vi "adsorption_rig_main.vi"() -> ()   [LabVIEW 2020]
uses:
  adam5000_LLB/controls/adam-5000-serial-settings.ctl
  adam5000_LLB/controls/adam-5000-cmd-response.ctl
  adam5000_LLB/controls/state-enum.ctl
  adam5000_LLB/sub-vi/csv-file-logging/filepath-selection.ctl
  adam5000_LLB/controls/adam-5000-all-chassis-data.ctl
  adam5000_LLB/controls/adam-5000-all-module-datas.ctl
  adam5000_LLB/controls/digital-output-cluster.ctl
  adam5000_LLB/controls/digitial-input-cluster.ctl
  adam5000_LLB/controls/analog-output-cluster.ctl
  adam5000_LLB/controls/analog-input-cluster.ctl
  adam5000_LLB/controls/thermocouple-input-cluster.ctl
  adam5000_LLB/controls/adam-5000-chassis-cmd-ack.ctl
  adam5000_LLB/controls/adam-5000-chassis-module-types.ctl
  adam5000_LLB/controls/adam-5000-DO-user-input.ctl
  adam5000_LLB/controls/adam-5000-status-indicator-references.ctl
panel:
  in  "Reset LD":bool
  out "longest delay":u32
  out "Next Log Event mS":u32
  in  "Tab Control":enum32{"System", "Settings"}(tab)
  in  "Flow 4":dbl
  in  "Flow 3":dbl
  in  "Flow 2":dbl
  in  "Flow 1":dbl
  in  "V9: EP1":bool
  in  "V12: EP4":bool
  in  "V10: EP2":bool
  in  "V11: EP3":bool
  in  "V15: \nRecirculation":bool
  in  "V14: HR2":bool
  out "TC9":dbl
  in  "V13: HR1":bool
  out "TC8":dbl
  in  "V8: In4":bool
  out "TC1":dbl
  out "TC2":dbl
  out "TC3":dbl
  out "TC4":dbl
  out "TC5":dbl
  out "TC6":dbl
  out "TC7":dbl
  out "TC10":dbl
  out "TC11":dbl
  out "TC12":dbl
  in  "V1: Ex1":bool
  in  "V2: Ex2":bool
  in  "V4: Ex4":bool
  in  "V5: In1":bool
  in  "V6: In2":bool
  in  "V7: In3":bool
  out "P1: Condenser":dbl
  out "P2: Adsorber 2":dbl
  out "P3: Adsorber 1":dbl
  out "P4: Evaporator":dbl
  in  "V3: Ex3":bool
  in  "Additional CSV Data Heading":string="Flow1,Flow2,Flow3,Flow4"
  in  "Chassis Settings":T1={"VISA resource name"="COM4", "baud rate (19200)"=19200, "Chassis ID"=1}
  in  "Log Filepath Selection":T2={"Log Filepath Source"=enum."Application Relative (Auto)", "Log File Path (Manual)"=path "C:/Users/iwheard/Documents/0000-labview/adam5000-generic-controller/data", "Log File Folder Name"="data", "log file name"="log", "Include Date in Filename"=TRUE, "Include Time in Filename"=TRUE}
  out "Log Filepath":path
  out "log start time":u32
  out "log-elapsed time":dbl format="%.2f"
  in  "CSV Data Headings":string="time (s),T1,T2,T3,T4,T5,T6,T7,T8,T9,T10,T11,T12,P1,P2,P3,P4"
  out "Logged Data String":string
  out "error":errorcluster
  out "Hz":dbl format="%_3g"
  in  "Sample Rate (Hz)":dbl=1.0 min=0.0001 max=4.0 format="%#_4g"
  out "File Open":bool
  out "Logging Active":bool
  out "Error Detected":bool
  in  "Reset":bool
  out "ADAM Connected":bool
  in  "Stop ADAM":bool
  in  "Start Logging":bool
  out "Program State":T3
  in  "Start ADAM":bool
  out "cmd-response":T5
  out "Status Indicators":T6
  in  "Debug Mode":bool
  out "Loop Time (mS)":u32
  out "Loop Counter":i32
  in  "exit":bool
  # "Adsorption Rig 2025"
  # "Built By: \nImogen Heard"
  # "Cold"
  # "Ambient"
  # "Hot"
  # "NV-002"
  # "NV-001"
  # "NV-004"
  # "Flow 4"
  # "Flow 1"
  # "Flow 2"
  # "NV-003"
  # "Flow 3"
  # "Condenser"
  # "Adsorber 1"
  # "Adsorber 2"
  # "Evaporator"
  # "Flow Meter Inputs"
  # "Pressure Sensors"
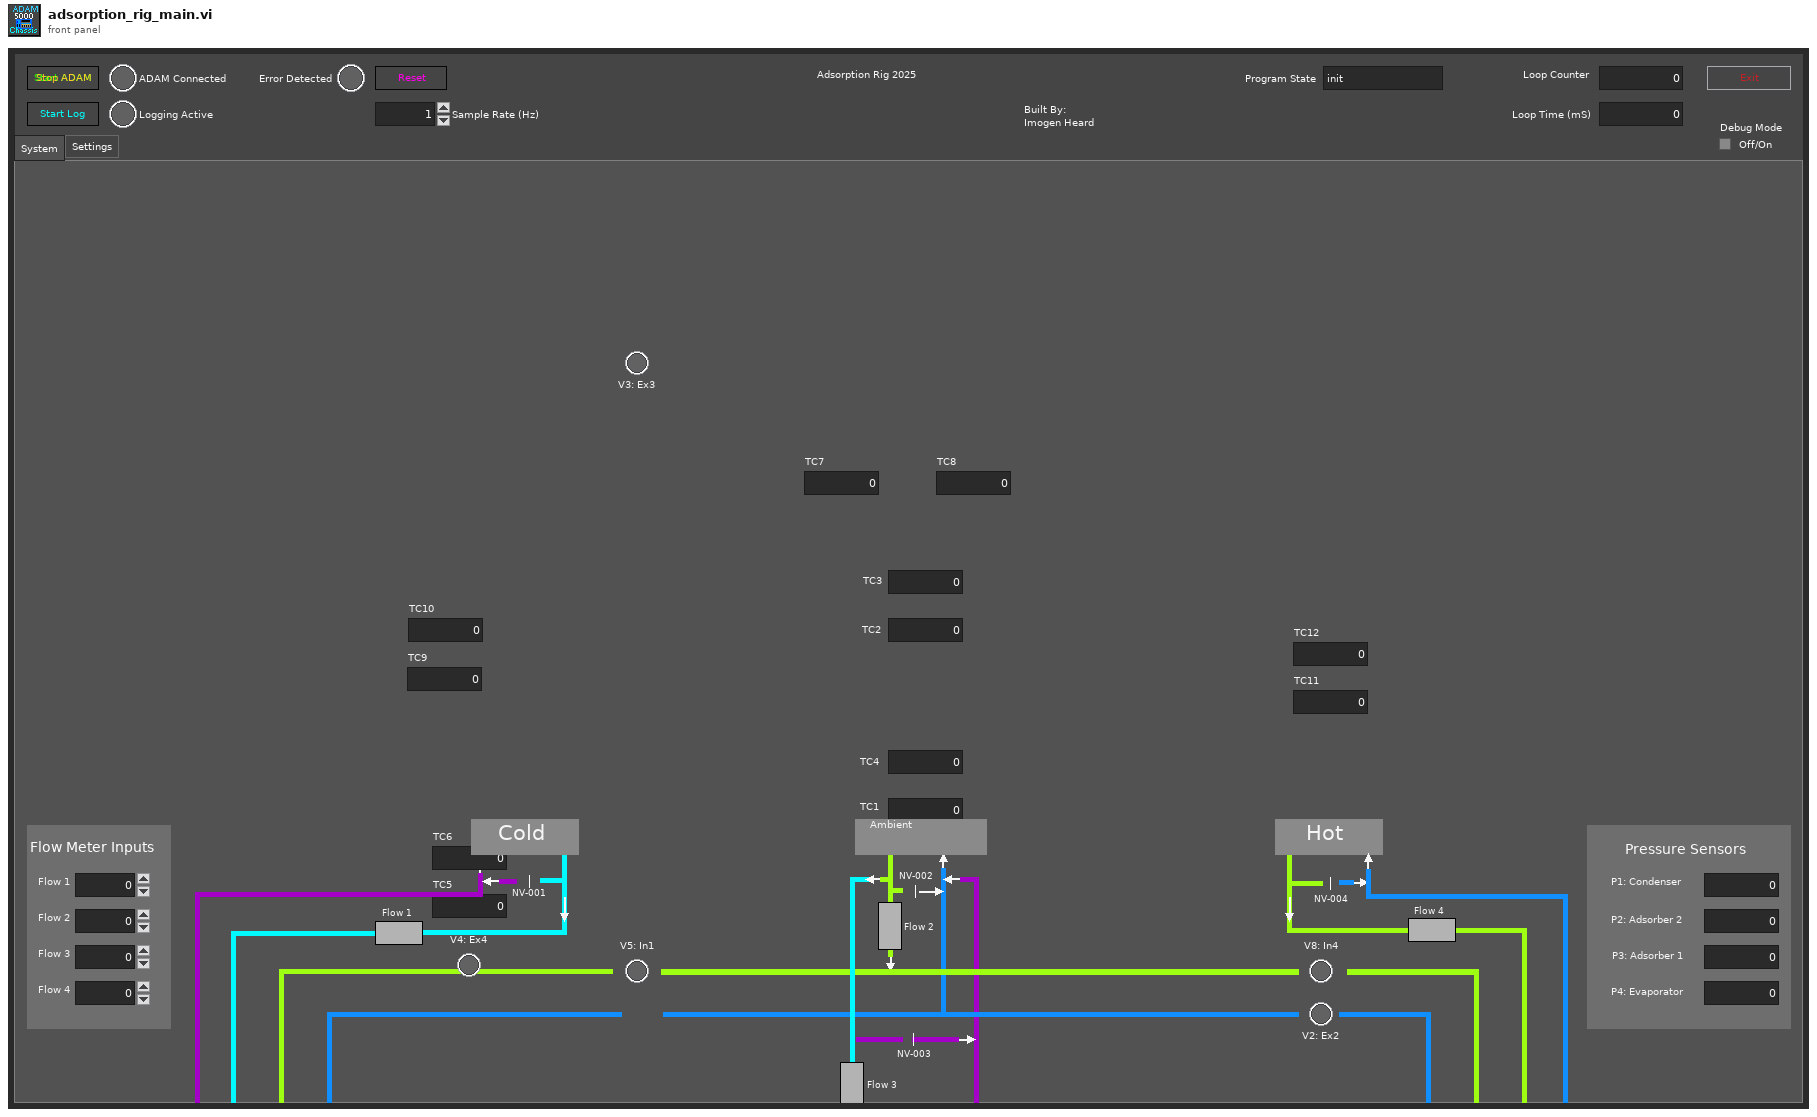
[diagram p1: front panel]
types:
  T1 = typedef "adam-5000-serial-settings.ctl" = cluster{"VISA resource name":refnum<visa-resource-name>, "baud rate (19200)":u32, "Chassis ID":u8}
  T2 = typedef "filepath-selection.ctl" = cluster{"Log Filepath Source":enum16{"Application Relative (Auto)", "VI Relative (Auto)", "Complete Path (Manual)"}, "Log File Path (Manual)":path, "Log File Folder Name":string, "log file name":string, "Include Date in Filename":bool, "Include Time in Filename":bool}
  T3 = typedef "state-enum.ctl" = enum16{"init", "wait", "manual", "start", "run", "reset", "stop", "exit"}
  T4 = typedef "adam-5000-cmd-response.ctl" = cluster{"cmd string":string, "response":string}
  T5 = cluster{"cmd-response:0":T4, "cmd-response:1":T4, "cmd-response:2":T4, "cmd-response:3":T4, "cmd-response:4":T4, "cmd-response:5":T4, "cmd-response:6":T4, "cmd-response:7":T4}
  T6 = cluster{"status-indicator:0":cluster{"Sampling":bool, "Ack":bool}, "status-indicator:1":cluster{"Sampling":bool, "Ack":bool}, "status-indicator:2":cluster{"Sampling":bool, "Ack":bool}, "status-indicator:3":cluster{"Sampling":bool, "Ack":bool}, "status-indicator:4":cluster{"Sampling":bool, "Ack":bool}, "status-indicator:5":cluster{"Sampling":bool, "Ack":bool}, "status-indicator:6":cluster{"Sampling":bool, "Ack":bool}, "status-indicator:7":cluster{"Sampling":bool, "Ack":bool}}
  T7 = enum16{"Digital Output", "Digital Input", "Analog Output", "Analog Input", "Thermocouple", "Power Relay", "empty"}
  T8 = typedef "adam-5000-chassis-module-types.ctl" = cluster{"Slot 0: Module Type":enum16{"Digital Output", "Digital Input", "Analog Output", "Analog Input", "Thermocouple", "Power Relay", "empty"}, "Slot 1: Module Type":enum16{"Digital Output", "Digital Input", "Analog Output", "Analog Input", "Thermocouple", "Power Relay", "empty"}, "Slot 2: Module Type":enum16{"Digital Output", "Digital Input", "Analog Output", "Analog Input", "Thermocouple", "Power Relay", "empty"}, "Slot 3: Module Type":enum16{"Digital Output", "Digital Input", "Analog Output", "Analog Input", "Thermocouple", "Power Relay", "empty"}, "Slot 4: Module Type":enum16{"Digital Output", "Digital Input", "Analog Output", "Analog Input", "Thermocouple", "Power Relay", "empty"}, "Slot 5: Module Type":enum16{"Digital Output", "Digital Input", "Analog Output", "Analog Input", "Thermocouple", "Power Relay", "empty"}, "Slot 6: Module Type":enum16{"Digital Output", "Digital Input", "Analog Output", "Analog Input", "Thermocouple", "Power Relay", "empty"}, "Slot 7: Module Type":enum16{"Digital Output", "Digital Input", "Analog Output", "Analog Input", "Thermocouple", "Power Relay", "empty"}}
  T9 = typedef "adam-5000-chassis-cmd-ack.ctl" = cluster{"cmd-response:0":T4, "cmd-response:1":T4, "cmd-response:2":T4, "cmd-response:3":T4, "cmd-response:4":T4, "cmd-response:5":T4, "cmd-response:6":T4, "cmd-response:7":T4}
  T10 = typedef "adam-5000-all-chassis-data.ctl" = cluster{"slot:0":T11, "slot:1":T11, "slot:2":T11, "slot:3":T11, "slot:4":T11, "slot:5":T11, "slot:6":T11, "slot:7":T11}
  T11 = typedef "adam-5000-all-module-datas.ctl" = cluster{"Digital Outputs":T12, "Digital Inputs":T13, "Analog Outputs":T14, "Analog Inputs":T15, "Thermocouple Inputs (degC)":T16}
  T12 = typedef "digital-output-cluster.ctl" = cluster{"DO0":bool, "DO1":bool, "DO2":bool, "DO3":bool, "DO4":bool, "DO5":bool, "DO6":bool, "DO7":bool}
  T13 = typedef "digitial-input-cluster.ctl" = cluster{"DI0":bool, "DI1":bool, "DI2":bool, "DI3":bool, "DI4":bool, "DI5":bool, "DI6":bool, "DI7":bool}
  T14 = typedef "analog-output-cluster.ctl" = cluster{"AO0":dbl, "AO1":dbl, "AO2":dbl, "AO3":dbl}
  T15 = typedef "analog-input-cluster.ctl" = cluster{"AI0":dbl, "AI1":dbl, "AI2":dbl, "AI3":dbl, "AI4":dbl, "AI5":dbl, "AI6":dbl, "AI7":dbl}
  T16 = typedef "thermocouple-input-cluster.ctl" = cluster{"TC0":dbl, "TC1":dbl, "TC2":dbl, "TC3":dbl, "TC4":dbl, "TC5":dbl, "TC6":dbl}
  T17 = enum8{"Enabled", "Disabled", "Disabled and Grayed Out"}
  T18 = typedef "adam-5000-status-indicator-references.ctl" = cluster{"status-indicator:0":refnum<vi>, "status-indicator:1":refnum<vi>, "status-indicator:2":refnum<vi>, "status-indicator:3":refnum<vi>, "status-indicator:4":refnum<vi>, "status-indicator:5":refnum<vi>, "status-indicator:6":refnum<vi>, "status-indicator:7":refnum<vi>}
  T19 = typedef "adam-5000-DO-user-input.ctl" = cluster{"0:Digital Outputs":T12, "1:Digital Outputs":T12, "2:Digital Outputs":T12, "3:Digital Outputs":T12, "4:Digital Outputs":T12, "5:Digital Outputs":T12, "6:Digital Outputs":T12, "7:Digital Outputs":T12}
  T20 = cluster{"V1: Ex1":bool, "V2: Ex2":bool, "V3: Ex3":bool, "V4: Ex4":bool, "V5: In1":bool, "V6: In2":bool, "V7: In3":bool, "V8: In4":bool}
  T21 = cluster{"V9: EP1":bool, "V10: EP2":bool, "V11: EP3":bool, "V12: EP4":bool, "V13: HR1":bool, "V14: HR2":bool, "V15: \nRecirculation":bool, "V9: EP1":bool}
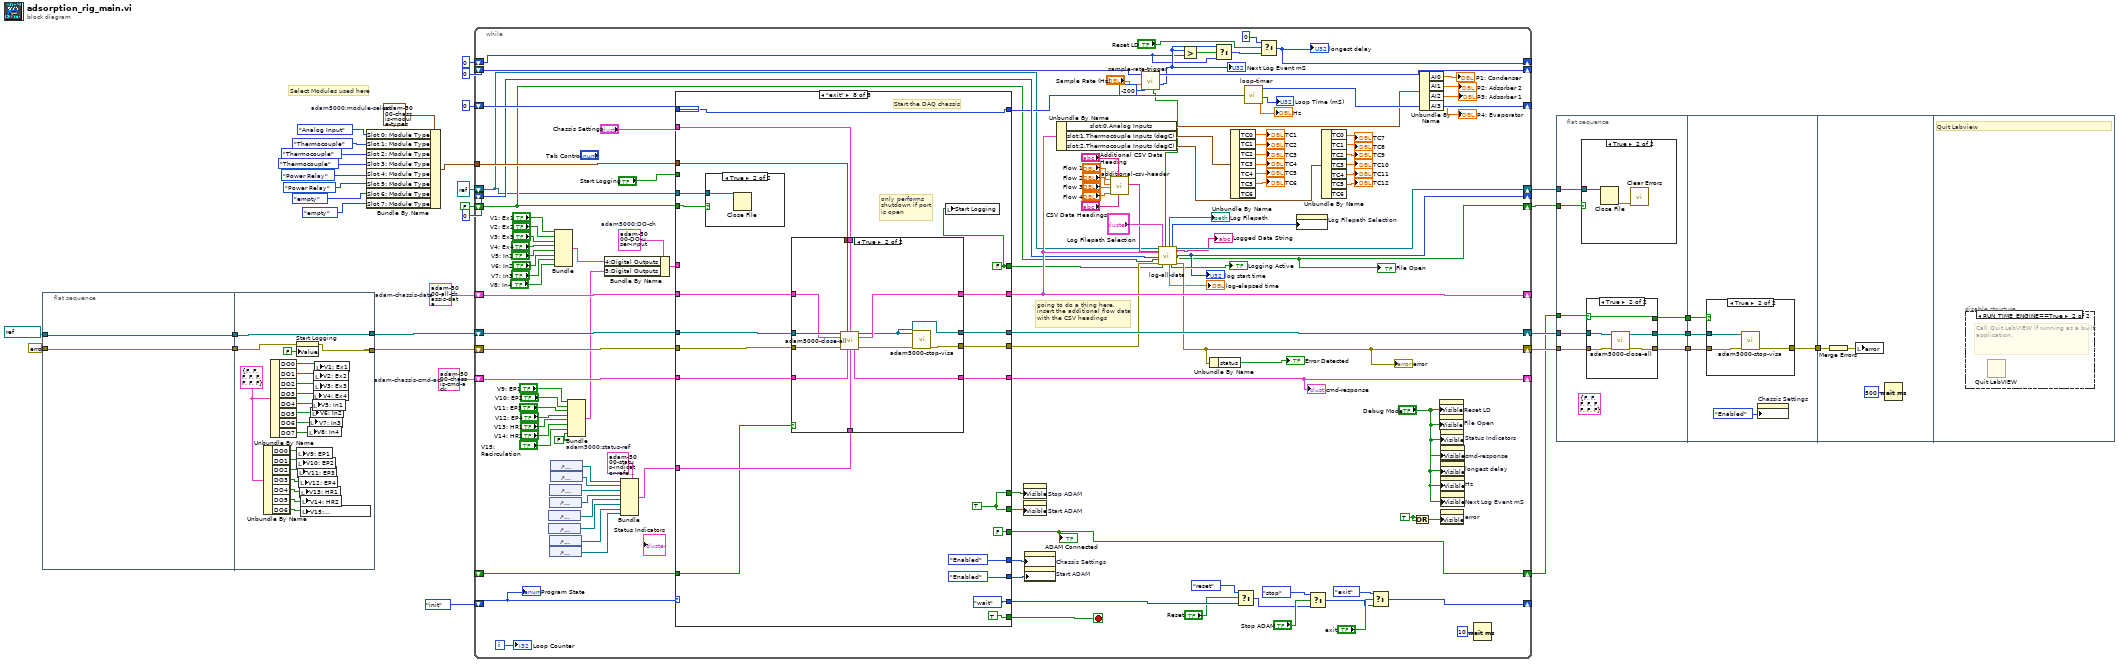
[diagram p0: block diagram]
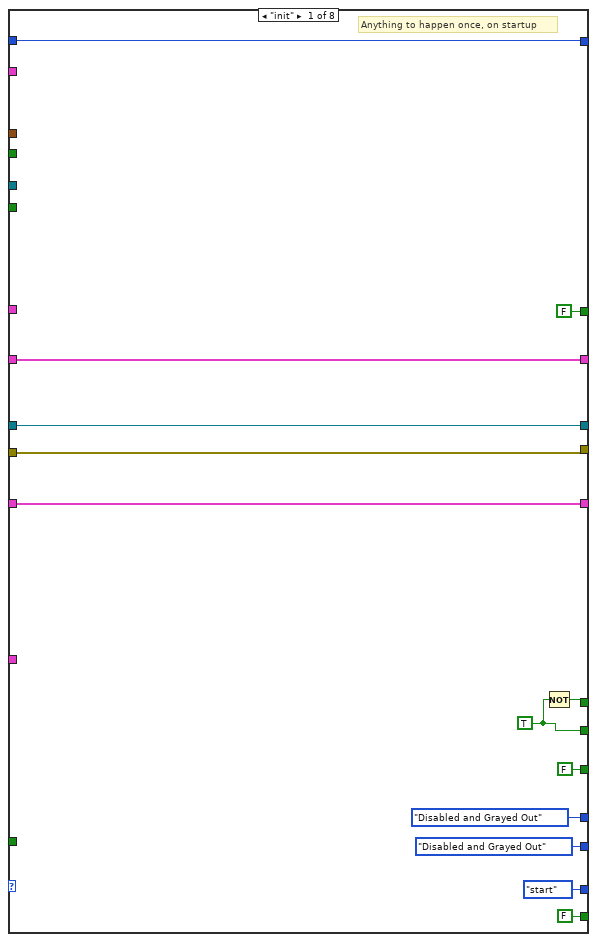
[diagram p6: hidden frame]
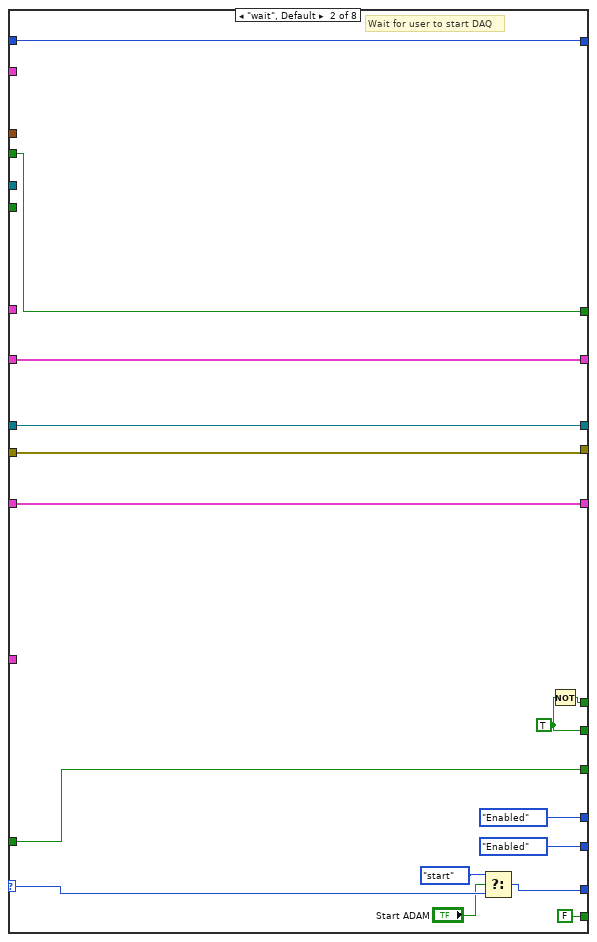
[diagram p7: hidden frame]
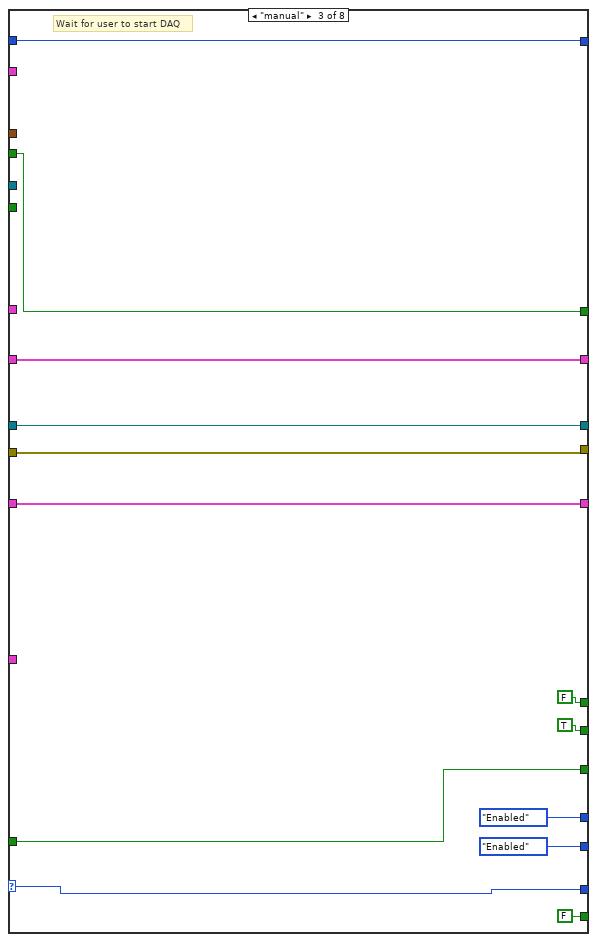
[diagram p8: hidden frame]
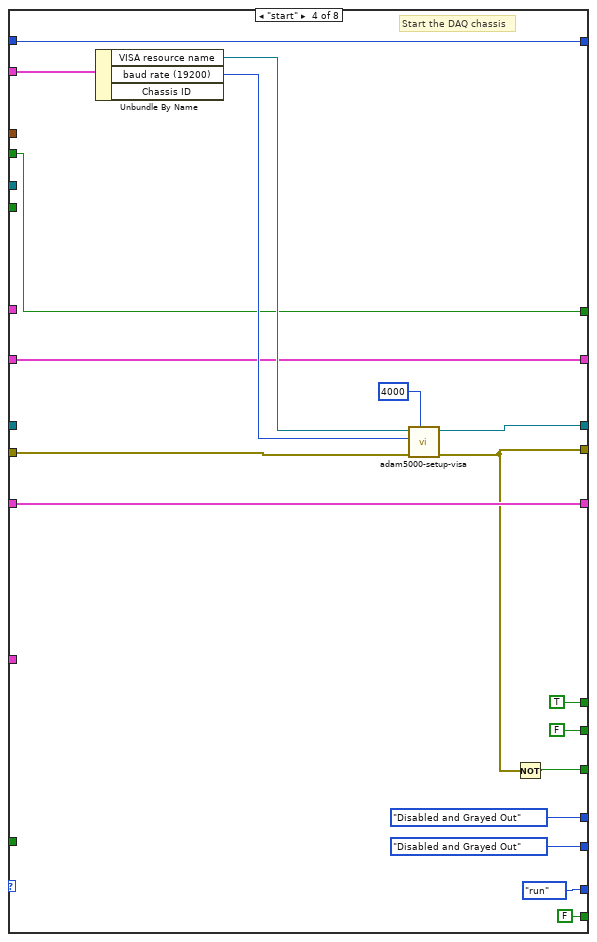
[diagram p9: hidden frame]
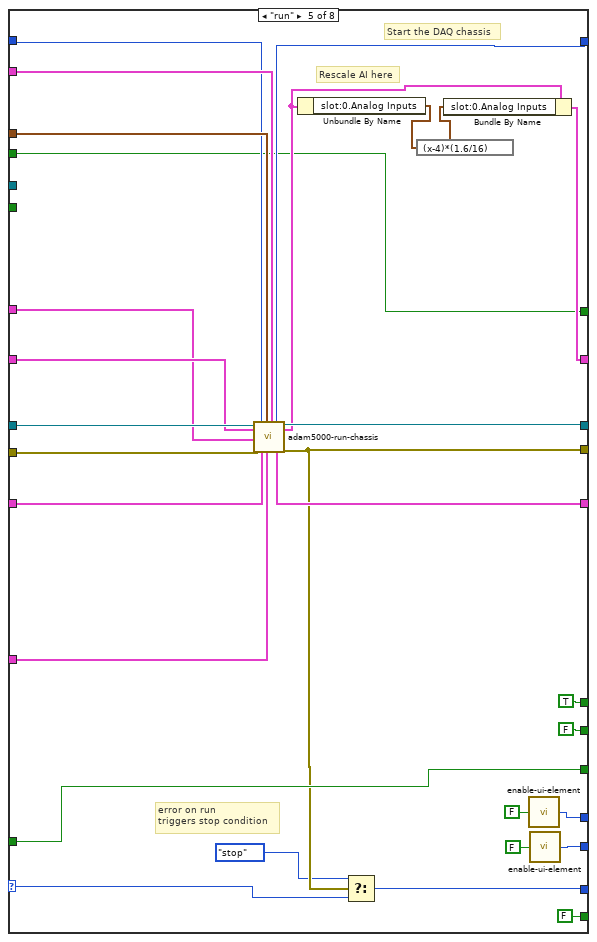
[diagram p10: hidden frame]
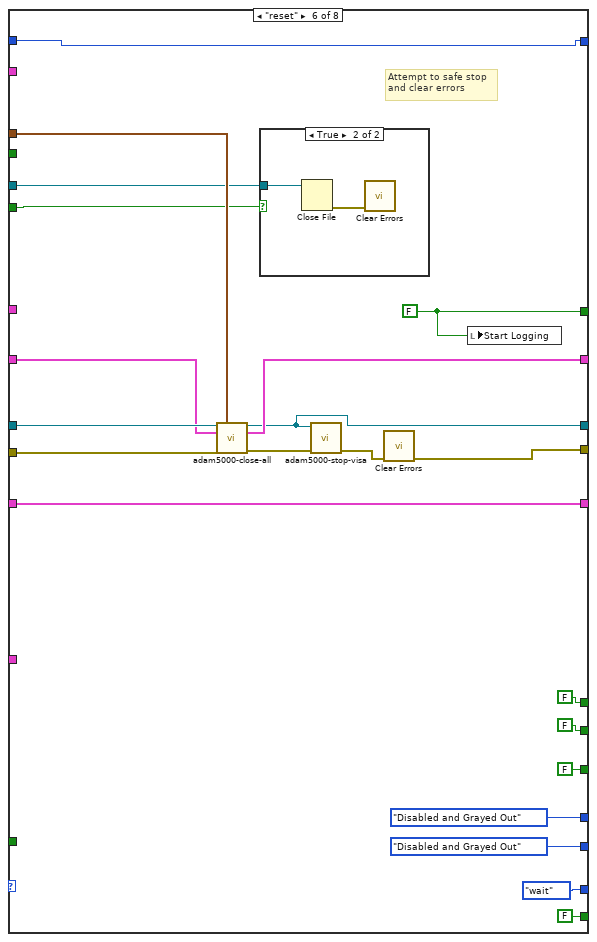
[diagram p11: hidden frame]
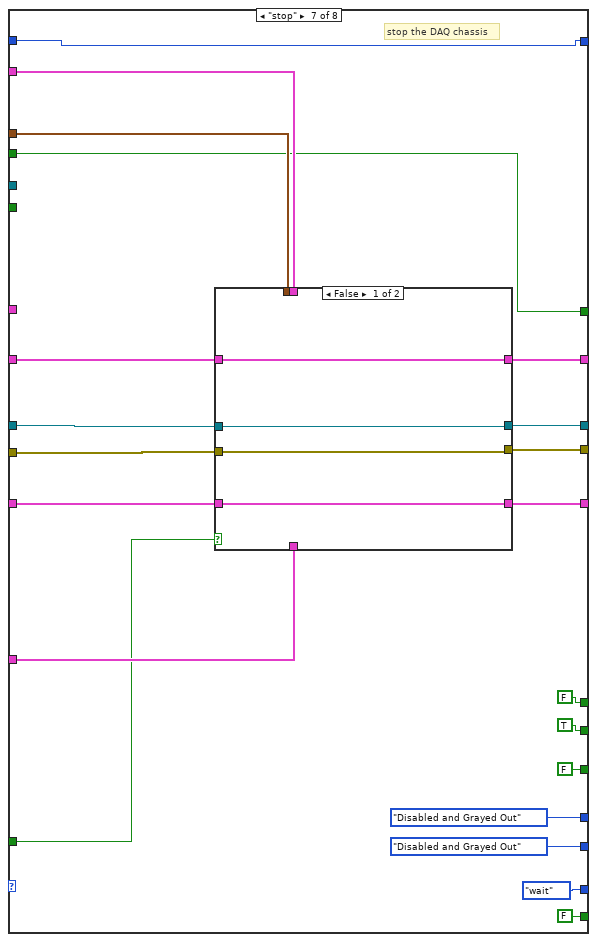
[diagram p13: hidden frame]
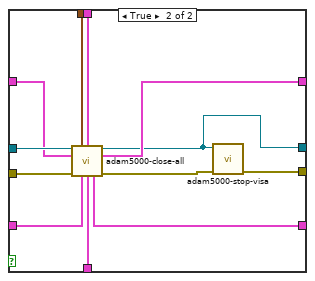
[diagram p14: hidden frame]
diagram:
  w26 = T8 {"Slot 0: Module Type"=enum."Digital Output", "Slot 1: Module Type"=enum."Digital Output", "Slot 2: Module Type"=enum."Digital Output", "Slot 3: Module Type"=enum."Digital Output", "Slot 4: Module Type"=enum."Digital Output", "Slot 5: Module Type"=enum."Digital Output", "Slot 6: Module Type"=enum."Digital Output", "Slot 7: Module Type"=enum."Digital Output"}  # adam5000:module-select
  w31 = T9 {"cmd-response:0"={"cmd string"="", "response"=""}, "cmd-response:1"={"cmd string"="", "response"=""}, "cmd-response:2"={"cmd string"="", "response"=""}, "cmd-response:3"={"cmd string"="", "response"=""}, "cmd-response:4"={"cmd string"="", "response"=""}, "cmd-response:5"={"cmd string"="", "response"=""}, "cmd-response:6"={"cmd string"="", "response"=""}, "cmd-response:7"={"cmd string"="", "response"=""}}  # adam-chassis-cmd-ack
  w32 = T10 {"slot:0"={"Digital Outputs"={"DO0"=FALSE, "DO1"=FALSE, "DO2"=FALSE, "DO3"=FALSE, "DO4"=FALSE, "DO5"=FALSE, "DO6"=FALSE, "DO7"=FALSE}, "Digital Inputs"={"DI0"=FALSE, "DI1"=FALSE, "DI2"=FALSE, "DI3"=FALSE, "DI4"=FALSE, "DI5"=FALSE, "DI6"=FALSE, "DI7"=FALSE}, "Analog Outputs"={"AO0"=0.0, "AO1"=0.0, "AO2"=0.0, "AO3"=0.0}, "Analog Inputs"={"AI0"=0.0, "AI1"=0.0, "AI2"=0.0, "AI3"=0.0, "AI4"=0.0, "AI5"=0.0, "AI6"=0.0, "AI7"=0.0}, "Thermocouple Inputs (degC)"={"TC0"=0.0, "TC1"=0.0, "TC2"=0.0, "TC3"=0.0, "TC4"=0.0, "TC5"=0.0, "TC6"=0.0}}, "slot:1"={"Digital Outputs"={"DO0"=FALSE, "DO1"=FALSE, "DO2"=FALSE, "DO3"=FALSE, "DO4"=FALSE, "DO5"=FALSE, "DO6"=FALSE, "DO7"=FALSE}, "Digital Inputs"={"DI0"=FALSE, "DI1"=FALSE, "DI2"=FALSE, "DI3"=FALSE, "DI4"=FALSE, "DI5"=FALSE, "DI6"=FALSE, "DI7"=FALSE}, "Analog Outputs"={"AO0"=0.0, "AO1"=0.0, "AO2"=0.0, "AO3"=0.0}, "Analog Inputs"={"AI0"=0.0, "AI1"=0.0, "AI2"=0.0, "AI3"=0.0, "AI4"=0.0, "AI5"=0.0, "AI6"=0.0, "AI7"=0.0}, "Thermocouple Inputs (degC)"={"TC0"=0.0, "TC1"=0.0, "TC2"=0.0, "TC3"=0.0, "TC4"=0.0, "TC5"=0.0, "TC6"=0.0}}, "slot:2"={"Digital Outputs"={"DO0"=FALSE, "DO1"=FALSE, "DO2"=FALSE, "DO3"=FALSE, "DO4"=FALSE, "DO5"=FALSE, "DO6"=FALSE, "DO7"=FALSE}, "Digital Inputs"={"DI0"=FALSE, "DI1"=FALSE, "DI2"=FALSE, "DI3"=FALSE, "DI4"=FALSE, "DI5"=FALSE, "DI6"=FALSE, "DI7"=FALSE}, "Analog Outputs"={"AO0"=0.0, "AO1"=0.0, "AO2"=0.0, "AO3"=0.0}, "Analog Inputs"={"AI0"=0.0, "AI1"=0.0, "AI2"=0.0, "AI3"=0.0, "AI4"=0.0, "AI5"=0.0, "AI6"=0.0, "AI7"=0.0}, "Thermocouple Inputs (degC)"={"TC0"=0.0, "TC1"=0.0, "TC2"=0.0, "TC3"=0.0, "TC4"=0.0, "TC5"=0.0, "TC6"=0.0}}, "slot:3"={"Digital Outputs"={"DO0"=FALSE, "DO1"=FALSE, "DO2"=FALSE, "DO3"=FALSE, "DO4"=FALSE, "DO5"=FALSE, "DO6"=FALSE, "DO7"=FALSE}, "Digital Inputs"={"DI0"=FALSE, "DI1"=FALSE, "DI2"=FALSE, "DI3"=FALSE, "DI4"=FALSE, "DI5"=FALSE, "DI6"=FALSE, "DI7"=FALSE}, "Analog Outputs"={"AO0"=0.0, "AO1"=0.0, "AO2"=0.0, "AO3"=0.0}, "Analog Inputs"={"AI0"=0.0, "AI1"=0.0, "AI2"=0.0, "AI3"=0.0, "AI4"=0.0, "AI5"=0.0, "AI6"=0.0, "AI7"=0.0}, "Thermocouple Inputs (degC)"={"TC0"=0.0, "TC1"=0.0, "TC2"=0.0, "TC3"=0.0, "TC4"=0.0, "TC5"=0.0, "TC6"=0.0}}, "slot:4"={"Digital Outputs"={"DO0"=FALSE, "DO1"=FALSE, "DO2"=FALSE, "DO3"=FALSE, "DO4"=FALSE, "DO5"=FALSE, "DO6"=FALSE, "DO7"=FALSE}, "Digital Inputs"={"DI0"=FALSE, "DI1"=FALSE, "DI2"=FALSE, "DI3"=FALSE, "DI4"=FALSE, "DI5"=FALSE, "DI6"=FALSE, "DI7"=FALSE}, "Analog Outputs"={"AO0"=0.0, "AO1"=0.0, "AO2"=0.0, "AO3"=0.0}, "Analog Inputs"={"AI0"=0.0, "AI1"=0.0, "AI2"=0.0, "AI3"=0.0, "AI4"=0.0, "AI5"=0.0, "AI6"=0.0, "AI7"=0.0}, "Thermocouple Inputs (degC)"={"TC0"=0.0, "TC1"=0.0, "TC2"=0.0, "TC3"=0.0, "TC4"=0.0, "TC5"=0.0, "TC6"=0.0}}, "slot:5"={"Digital Outputs"={"DO0"=FALSE, "DO1"=FALSE, "DO2"=FALSE, "DO3"=FALSE, "DO4"=FALSE, "DO5"=FALSE, "DO6"=FALSE, "DO7"=FALSE}, "Digital Inputs"={"DI0"=FALSE, "DI1"=FALSE, "DI2"=FALSE, "DI3"=FALSE, "DI4"=FALSE, "DI5"=FALSE, "DI6"=FALSE, "DI7"=FALSE}, "Analog Outputs"={"AO0"=0.0, "AO1"=0.0, "AO2"=0.0, "AO3"=0.0}, "Analog Inputs"={"AI0"=0.0, "AI1"=0.0, "AI2"=0.0, "AI3"=0.0, "AI4"=0.0, "AI5"=0.0, "AI6"=0.0, "AI7"=0.0}, "Thermocouple Inputs (degC)"={"TC0"=0.0, "TC1"=0.0, "TC2"=0.0, "TC3"=0.0, "TC4"=0.0, "TC5"=0.0, "TC6"=0.0}}, "slot:6"={"Digital Outputs"={"DO0"=FALSE, "DO1"=FALSE, "DO2"=FALSE, "DO3"=FALSE, "DO4"=FALSE, "DO5"=FALSE, "DO6"=FALSE, "DO7"=FALSE}, "Digital Inputs"={"DI0"=FALSE, "DI1"=FALSE, "DI2"=FALSE, "DI3"=FALSE, "DI4"=FALSE, "DI5"=FALSE, "DI6"=FALSE, "DI7"=FALSE}, "Analog Outputs"={"AO0"=0.0, "AO1"=0.0, "AO2"=0.0, "AO3"=0.0}, "Analog Inputs"={"AI0"=0.0, "AI1"=0.0, "AI2"=0.0, "AI3"=0.0, "AI4"=0.0, "AI5"=0.0, "AI6"=0.0, "AI7"=0.0}, "Thermocouple Inputs (degC)"={"TC0"=0.0, "TC1"=0.0, "TC2"=0.0, "TC3"=0.0, "TC4"=0.0, "TC5"=0.0, "TC6"=0.0}}, "slot:7"={"Digital Outputs"={"DO0"=FALSE, "DO1"=FALSE, "DO2"=FALSE, "DO3"=FALSE, "DO4"=FALSE, "DO5"=FALSE, "DO6"=FALSE, "DO7"=FALSE}, "Digital Inputs"={"DI0"=FALSE, "DI1"=FALSE, "DI2"=FALSE, "DI3"=FALSE, "DI4"=FALSE, "DI5"=FALSE, "DI6"=FALSE, "DI7"=FALSE}, "Analog Outputs"={"AO0"=0.0, "AO1"=0.0, "AO2"=0.0, "AO3"=0.0}, "Analog Inputs"={"AI0"=0.0, "AI1"=0.0, "AI2"=0.0, "AI3"=0.0, "AI4"=0.0, "AI5"=0.0, "AI6"=0.0, "AI7"=0.0}, "Thermocouple Inputs (degC)"={"TC0"=0.0, "TC1"=0.0, "TC2"=0.0, "TC3"=0.0, "TC4"=0.0, "TC5"=0.0, "TC6"=0.0}}}  # adam-chassis-data
  # "Select Modules used here"
  n1 = flat-sequence {
    tunnel: errorcluster {"status"=FALSE, "code"=0, "source"=""} ("error in") -> [w35]
    tunnel: refnum<visa-resource-name> "COM8" ("VISA Refnum out") -> [w36]
    tunnel: [w36] -> w8
    tunnel: [w35] -> w7
    tunnel: [w55] -> w15
    tunnel: [w53] -> w13
    tunnel: w8 -> [w55]
    tunnel: w7 -> [w54]
    frame #0 {
    }
    frame #1 {
      w44 = T12 {"DO0"=FALSE, "DO1"=FALSE, "DO2"=FALSE, "DO3"=FALSE, "DO4"=FALSE, "DO5"=FALSE, "DO6"=FALSE, "DO7"=FALSE} ("5:Digital Outputs")
      n2 = Unbundle By Name(w44) -> ("DO0"=w43:bool, "DO1"=w42:bool, "DO2"=w41:bool, "DO3"=w40:bool, "DO4"=w39:bool, "DO5"=w38:bool, "DO6"=w37:bool)
      n3 = Unbundle By Name(w44) -> ("DO0"=w52:bool, "DO1"=w51:bool, "DO2"=w50:bool, "DO3"=w49:bool, "DO4"=w48:bool, "DO5"=w47:bool, "DO6"=w46:bool, "DO7"=w45:bool)
      n4 = property on="Start Logging" class="Bool (strict)"(error in=w54, "Value"=FALSE ("Start Logging")) -> (error out=w53:errorcluster)  [unwired: 1 in, 1 out]
      n5 = local write "V9: EP1"(w43) -> ()
      n6 = local write "V10: EP2"(w42) -> ()
      n7 = local write "V11: EP3"(w41) -> ()
      n8 = local write "V12: EP4"(w40) -> ()
      n9 = local write "V13: HR1"(w39) -> ()
      n10 = local write "V14: HR2"(w38) -> ()
      n11 = local write "V15: \nRecirculation"(w37) -> ()
      n12 = local write "V8: In4"(w45) -> ()
      n13 = local write "V7: In3"(w46) -> ()
      n14 = local write "V6: In2"(w47) -> ()
      n15 = local write "V5: In1"(w48) -> ()
      n16 = local write "V4: Ex4"(w49) -> ()
      n17 = local write "V2: Ex2"(w51) -> ()
      n18 = local write "V3: Ex3"(w50) -> ()
      n19 = local write "V1: Ex1"(w52) -> ()
    }
  }
  n20 = Bundle By Name(cluster=w26, "Slot 0: Module Type"=T7."Analog Input", "Slot 1: Module Type"=T7."Thermocouple", "Slot 2: Module Type"=T7."Thermocouple" ("Slot 1: Module Type"), "Slot 3: Module Type"=T7."Thermocouple" ("Slot 1: Module Type"), "Slot 4: Module Type"=T7."Power Relay" ("Slot 1: Module Type"), "Slot 5: Module Type"=T7."Power Relay" ("Slot 1: Module Type"), "Slot 6: Module Type"=T7."empty" ("Slot 1: Module Type"), "Slot 7: Module Type"=T7."empty" ("Slot 1: Module Type")) -> (w17:T8)
  n21 = while {
    shift-right: [w156] -> _
    shift-left: state-enum."init" ("state-enum") -> [w139]
    shift-right: [w123] -> _
    shift-left: u32 0 ("loop-time-out") -> [w161]
    shift-right: [w148] -> w30
    shift-left: w15 -> [w164]
    shift-right: [w128] -> w29
    shift-left: w13 -> [w163]
    shift-right: [w130] -> _
    shift-left: w32 -> [w160]
    shift-right: [w141] -> _
    shift-left: w31 -> [w158]
    shift-right: [w146] -> w11
    shift-left: _ -> [w147]
    tunnel: w17 -> [w140]
    shift-right: [w119] -> w10
    shift-left: FALSE ("file open?") -> [w70]
    shift-right: [w120] -> _
    shift-left: u32 0 ("log-start-time(mS)") -> [w129]
    shift-right: [w133] -> w9
    shift-left: refnum<file> refnum ("log-file-bytestream") -> [w69]
    shift-right: [w73] -> _
    shift-left: u32 0 ("last-event-mS out") -> [w72]
    shift-right: [w61] -> _
    shift-left: u32 0 ("Elapsed Time mS") -> [w65]
    i -> [w178]
    stop <- w149 stop-if-true
    w167 = T18 {"status-indicator:0"=refnum, "status-indicator:1"=refnum, "status-indicator:2"=refnum, "status-indicator:3"=refnum, "status-indicator:4"=refnum, "status-indicator:5"=refnum, "status-indicator:6"=refnum, "status-indicator:7"=refnum}  # adam5000:status-ref
    w168 = T19 {"0:Digital Outputs"={"DO0"=FALSE, "DO1"=FALSE, "DO2"=FALSE, "DO3"=FALSE, "DO4"=FALSE, "DO5"=FALSE, "DO6"=FALSE, "DO7"=FALSE}, "1:Digital Outputs"={"DO0"=FALSE, "DO1"=FALSE, "DO2"=FALSE, "DO3"=FALSE, "DO4"=FALSE, "DO5"=FALSE, "DO6"=FALSE, "DO7"=FALSE}, "2:Digital Outputs"={"DO0"=FALSE, "DO1"=FALSE, "DO2"=FALSE, "DO3"=FALSE, "DO4"=FALSE, "DO5"=FALSE, "DO6"=FALSE, "DO7"=FALSE}, "3:Digital Outputs"={"DO0"=FALSE, "DO1"=FALSE, "DO2"=FALSE, "DO3"=FALSE, "DO4"=FALSE, "DO5"=FALSE, "DO6"=FALSE, "DO7"=FALSE}, "4:Digital Outputs"={"DO0"=FALSE, "DO1"=FALSE, "DO2"=FALSE, "DO3"=FALSE, "DO4"=FALSE, "DO5"=FALSE, "DO6"=FALSE, "DO7"=FALSE}, "5:Digital Outputs"={"DO0"=FALSE, "DO1"=FALSE, "DO2"=FALSE, "DO3"=FALSE, "DO4"=FALSE, "DO5"=FALSE, "DO6"=FALSE, "DO7"=FALSE}, "6:Digital Outputs"={"DO0"=FALSE, "DO1"=FALSE, "DO2"=FALSE, "DO3"=FALSE, "DO4"=FALSE, "DO5"=FALSE, "DO6"=FALSE, "DO7"=FALSE}, "7:Digital Outputs"={"DO0"=FALSE, "DO1"=FALSE, "DO2"=FALSE, "DO3"=FALSE, "DO4"=FALSE, "DO5"=FALSE, "DO6"=FALSE, "DO7"=FALSE}}  # adam5000:DO-ch
    w150 = TRUE ("Debug Mode")
    # "going to do a thing here,\ninsert the additional flow data \nwith the CSV headings"
    n22 = control-ref of="status-indicator:4"() -> (w172:refnum<vi>)
    n23 = control-ref of="status-indicator:5"() -> (w171:refnum<vi>)
    n24 = control-ref of="status-indicator:3"() -> (w173:refnum<vi>)
    n25 = control-ref of="status-indicator:6"() -> (w170:refnum<vi>)
    n26 = control-ref of="status-indicator:7"() -> (w169:refnum<vi>)
    n27 = control-ref of="status-indicator:2"() -> (w174:refnum<vi>)
    n28 = control-ref of="status-indicator:0"() -> (w176:refnum<vi>)
    n29 = control-ref of="status-indicator:1"() -> (w175:refnum<vi>)
    n30 = Bundle("V1: Ex1"="V1: Ex1", "V2: Ex2"="V2: Ex2", "V3: Ex3"="V3: Ex3", "V4: Ex4"="V4: Ex4", "V5: In1"="V5: In1", "V6: In2"="V6: In2", "V7: In3"="V7: In3", "V8: In4"="V8: In4") -> (w110:T20)  [unwired: 1 in]
    n31 = Bundle("V9: EP1"="V9: EP1", "V10: EP2"="V10: EP2", "V11: EP3"="V11: EP3", "V12: EP4"="V12: EP4", "V13: HR1"="V13: HR1", "V14: HR2"="V14: HR2", "V15: \nRecirculation"="V15: \nRecirculation", "V9: EP1"=FALSE) -> (w101:T21)  [unwired: 1 in]
    n32 = Bundle By Name(cluster=w168, "4:Digital Outputs"=w110, "5:Digital Outputs"=w101) -> (w159:T19)
    n33 = Bundle(cluster=w167, "status-indicator:0"=w176, "status-indicator:1"=w175, "status-indicator:2"=w174, "status-indicator:3"=w173, "status-indicator:4"=w172, "status-indicator:5"=w171, "status-indicator:6"=w170, "status-indicator:7"=w169) -> (w157:T18)
    n34 = case shown="\"exit\"" w139 {
      selector: w139 -> [_ w205 w216 _ w252 _ _ _]
      tunnel: [state-enum."start" ("state-enum") w206 w216 state-enum."run" ("state-enum") w253 state-enum."wait" ("state-enum") state-enum."wait" ("state-enum") state-enum."wait" ("state-enum")] -> w144
      tunnel: [T17."Disabled and Grayed Out" ("Disabled") T17."Enabled" ("Disabled") T17."Enabled" ("Disabled") T17."Disabled and Grayed Out" ("Disabled") w242 T17."Disabled and Grayed Out" ("Disabled") T17."Disabled and Grayed Out" ("Disabled") T17."Enabled" ("Disabled")] -> w166
      tunnel: [T17."Disabled and Grayed Out" ("Disabled") T17."Enabled" ("Disabled") T17."Enabled" ("Disabled") T17."Disabled and Grayed Out" ("Disabled") w240 T17."Disabled and Grayed Out" ("Disabled") T17."Disabled and Grayed Out" ("Disabled") T17."Enabled" ("Disabled")] -> w165
      tunnel: w164 -> [w188 w202 w218 _ w267 w279 w308 w346]
      tunnel: [w188 w202 w218 w236 w265 w273 w298 w334] -> w148
      tunnel: w163 -> [w187 w201 w217 w235 w266 w278 w307 w345]
      tunnel: [w187 w201 w217 w225 w251 w282 w297 w335] -> w127
      tunnel: "Chassis Settings" -> [_ _ _ w234 w264 _ w305 w343]
      tunnel: w140 -> [_ _ _ _ w263 w275 w306 w344]
      tunnel: w161 -> [w186 w199 w215 w229 w262 w284 w299 w337]
      tunnel: [w186 w199 w215 w229 w261 w284 w299 w337] -> w124
      tunnel: w160 -> [w185 w198 w214 w228 w260 w277 w304 w342]
      tunnel: w159 -> [_ _ _ _ w259 _ _ _]
      tunnel: w158 -> [w184 w197 w213 w227 w258 w283 w302 w340]
      tunnel: w157 -> [_ _ _ _ w257 _ w301 w339]
      tunnel: [w184 w197 w213 w227 w256 w283 w300 w338] -> w141
      tunnel: [w185 w198 w214 w228 w246 w276 w303 w341] -> w130
      tunnel: [FALSE FALSE FALSE FALSE FALSE FALSE FALSE TRUE] -> w149
      tunnel: [FALSE w195 w211 w224 w254 FALSE FALSE FALSE] -> w146
      tunnel: w147 -> [_ w195 w211 _ w254 _ w294 w332]
      tunnel: [w181 w193 TRUE ("Visible") FALSE ("Visible") FALSE ("Visible") FALSE ("Visible") TRUE ("Visible") w331] -> w138
      tunnel: [w180 w194 FALSE ("Visible") TRUE ("Visible") TRUE ("Visible") FALSE ("Visible") FALSE ("Visible") w331] -> w137
      tunnel: w70 -> [_ _ _ _ _ w270 _ w329]
      tunnel: w69 -> [_ _ _ _ _ w269 _ w330]
      tunnel: "Start Logging" -> [_ w192 w208 w221 w239 _ w291 _]
      tunnel: [FALSE ("Start Logging") w192 w208 w221 w239 w268 w291 w328] -> w57
      frame "init" {
        w181 = TRUE ("Visible")
        # "Anything to happen once, on startup"
        n35 = Not(x=w181) -> (.not. x?=w180:bool)
      }
      frame "wait", Default {
        w193 = TRUE ("Visible")
        # "Wait for user to start DAQ"
        n36 = Select(t=state-enum."start" ("state-enum"), s="Start ADAM", f=w205) -> (s? t:f=w206:T3)
        n37 = Not(x=w193) -> (.not. x?=w194:bool)
      }
      frame "manual" {
        # "Wait for user to start DAQ"
      }
      frame "start" {
        # "Start the DAQ chassis"
        n38 = Unbundle By Name(w234) -> ("VISA resource name"=w233:refnum<visa-resource-name>, "baud rate (19200)"=w232:u32)  [unwired: 1 out]
        n39 = call "adam5000-setup-visa.vi"("timeout (10sec)"=u32 4000, "error in"=w235, "baud rate (19200)"=w232, "VISA Refnum in"=w233) -> ("error out"=w225:errorcluster, "VISA Refnum out"=w236:refnum<visa-resource-name>)  [unwired: 6 in]
        n40 = Not(x=w225) -> (.not. x?=w224:bool)
      }
      frame "run" {
        # "Rescale AI here"
        # "error on run\ntriggers stop condition"
        # "Start the DAQ chassis"
        n41 = call "adam5000-run-chassis.vi"("VISA Refnum In"=w267, "adam-chassis-all-data-in"=w260, "adam-chassis-all-DO-in"=w259, "error in"=w266, "loop-time-in"=w262, "adam-chassis-cmd-response-in"=w258, "adam-chassis-module-select-in"=w263, "adam5000:status-ref-in"=w257, "Chassis Settings"=w264) -> ("loop-time-out"=w261:u32, "adam-chassis-cmd-response-out"=w256:T9, "VISA Refnum Out"=w265:refnum<visa-resource-name>, "adam-chassis-all-data-out"=w247:T10, "error out"=w251:errorcluster)  [unwired: 5 in, 1 out]
        n42 = Unbundle By Name(w247) -> ("slot:0.Analog Inputs"=w245:T15)
        n43 = Select(t=state-enum."stop", s=w251, f=w252) -> (s? t:f=w253:T3)
        n44 = expression code="(x-4)*(1.6/16)"(w245) -> (w244:T15)
        n45 = Bundle By Name(cluster=w247, "slot:0.Analog Inputs"=w244) -> (w246:T10)
        n46 = call "enable-ui-element.vi"("Enable UI Element"=FALSE) -> ("UI Element State"=w242:T17)  [unwired: 8 in]
        n47 = call "enable-ui-element.vi"("Enable UI Element"=FALSE) -> ("UI Element State"=w240:T17)  [unwired: 8 in]
      }
      frame "reset" {
        w268 = FALSE ("Start Logging")
        # "Attempt to safe stop\nand clear errors"
        n48 = call "adam5000-close-all.vi"("VISA Refnum in"=w279, "adam5000:module-type-select"=w275, "adam5000:all-data-in"=w277, "error in (no error)"=w278) -> ("VISA Refnum out"=w273:refnum<visa-resource-name>, "adam5000:all-data-out"=w276:T10, "error out"=w280:errorcluster)  [unwired: 8 in, 1 out]
        n49 = case shown="True" w270 {
          tunnel: w269 -> [_ w290]
          frame False {
          }
          frame True {
            n50 = Close File(refnum=w290) -> (error out=w289:errorcluster)  [unwired: 1 in, 1 out]
            n51 = call <vilib>:"Clear Errors.vi"("error in (no error)"=w289) -> ()  [unwired: 5 in, 2 out]
          }
        }
        n52 = call "adam5000-stop-visa.vi"("error in (no error)"=w280, "VISA resource in"=w273) -> ("error out"=w274:errorcluster)  [unwired: 9 in]
        n53 = call <vilib>:"Clear Errors.vi"("error in (no error)"=w274) -> ("error out"=w282:errorcluster)  [unwired: 5 in, 1 out]
        n54 = local write "Start Logging"(w268) -> ()
      }
      frame "stop" {
        # "stop the DAQ chassis"
        n55 = case shown="False" w294 {
          tunnel: w308 -> [w313 w327]
          tunnel: w307 -> [w312 w326]
          tunnel: w306 -> [_ w325]
          tunnel: w305 -> [_ w324]
          tunnel: w304 -> [w315 w323]
          tunnel: [w315 w322] -> w303
          tunnel: w302 -> [w314 w321]
          tunnel: w301 -> [_ w320]
          tunnel: [w314 w319] -> w300
          tunnel: [w313 w318] -> w298
          tunnel: [w312 w316] -> w297
          frame False {
          }
          frame True {
            n56 = call "adam5000-close-all.vi"("VISA Refnum in"=w327, "adam5000:module-type-select"=w325, "Chassis Settings in"=w324, "adam5000:all-data-in"=w323, "error in (no error)"=w326, "adam-chassis-cmd-ack"=w321, "adam5000:status-ref"=w320) -> ("VISA Refnum out"=w318:refnum<visa-resource-name>, "adam5000:all-data-out"=w322:T10, "adam-chassis-cmd-response-out"=w319:T9, "error out"=w317:errorcluster)  [unwired: 5 in]
            n57 = call "adam5000-stop-visa.vi"("error in (no error)"=w317, "VISA resource in"=w318) -> ("error out"=w316:errorcluster)  [unwired: 9 in]
          }
        }
      }
      frame "exit" {
        w328 = FALSE ("Start Logging")
        w331 = TRUE ("Visible")
        # "only performs\nshutdown if port\nis open"
        # "Start the DAQ chassis"
        n58 = case shown="True" w329 {
          tunnel: w330 -> [_ w350]
          frame False {
          }
          frame True {
            n59 = Close File(refnum=w350) -> ()  [unwired: 1 in, 2 out]
          }
        }
        n60 = case shown="True" w332 {
          tunnel: w346 -> [w353 w366]
          tunnel: w345 -> [w352 w365]
          tunnel: w344 -> [_ w364]
          tunnel: w343 -> [_ w363]
          tunnel: w342 -> [w354 w362]
          tunnel: [w354 w361] -> w341
          tunnel: w340 -> [w351 w360]
          tunnel: w339 -> [_ w359]
          tunnel: [w351 w358] -> w338
          tunnel: [w352 w356] -> w335
          tunnel: [w353 w355] -> w334
          frame False {
          }
          frame True {
            n61 = call "adam5000-close-all.vi"("VISA Refnum in"=w366, "adam5000:module-type-select"=w364, "Chassis Settings in"=w363, "adam5000:all-data-in"=w362, "error in (no error)"=w365, "adam-chassis-cmd-ack"=w360, "adam5000:status-ref"=w359) -> ("VISA Refnum out"=w355:refnum<visa-resource-name>, "adam5000:all-data-out"=w361:T10, "adam-chassis-cmd-response-out"=w358:T9, "error out"=w357:errorcluster)  [unwired: 5 in]
            n62 = call "adam5000-stop-visa.vi"("error in (no error)"=w357, "VISA resource in"=w355) -> ("error out"=w356:errorcluster)  [unwired: 9 in]
          }
        }
        n63 = local write "Start Logging"(w328) -> ()
      }
    }
    "cmd-response" <- w141
    "ADAM Connected" <- w146
    n64 = property on="Stop ADAM" class="Bool"("Visible"=w137) -> ()  [unwired: 2 in, 2 out]
    n65 = property on="Start ADAM" class="Bool"("Visible"=w138) -> ()  [unwired: 2 in, 2 out]
    n66 = property on="Chassis Settings" class="Clust (strict)"("DisabledEnum"=w166) -> ()  [unwired: 2 in, 2 out]
    n67 = property on="Start ADAM" class="Bool"("DisabledEnum"=w165) -> ()  [unwired: 2 in, 2 out]
    n68 = Unbundle By Name(w130) -> ("slot:0.Analog Inputs"=w93:T15, "slot:1.Thermocouple Inputs (degC)"=w88:T16, "slot:2.Thermocouple Inputs (degC)"=w81:T16)
    n69 = call "additional-csv-header.vi"("CSV Data Headings"="CSV Data Headings", "Additional Text Heading"="Additional CSV Data Heading", "Flow 4"="Flow 4", "Flow 3"="Flow 3", "Flow 2"="Flow 2", "Flow 1"="Flow 1") -> ("new-csv-header"=w94:string)  [unwired: 5 in]
    n70 = call "sample-rate-trigger.vi"("last-event-mS in"=w72, "Sample Rate (Hz)"="Sample Rate (Hz)", "mS modifyer"=-200) -> ("triggered?"=w71:bool, "last-event-mS out"=w73:u32, "Elapsed Time mS"=w66:u32)  [unwired: 4 in, 1 out]
    "Next Log Event mS" <- w66
    n71 = call "log-all-data.vi"("log-file-byte-stream"=w69, "CSV Data Headings"=w94, "adam5000:all-data-in"=w130, "log-start-time(mS)"=w129, "file open?"=w70, "error in (no error)"=w127, "Log Filepath Selection"="Log Filepath Selection", "Start Logging"=w57, "Enable Log Trigger"=w71) -> ("appended path for log file"=→"Log Filepath":path, "log-elapsed time"=→"log-elapsed time":dbl, "log-filepath-enable-state"=w132:T17, "Start Logging"=→"Logging Active":bool, "log-file-bytestream"=w133:refnum<file>, "Logged Data String"=→"Logged Data String":string, "log-start-time(mS)"=w120:u32, "file open?"=w119:bool, "error out"=w128:errorcluster)  [unwired: 2 in]
    "error" <- w128
    "File Open" <- w119
    "log start time" <- w120
    n72 = Greater?(x=w66, y=w65) -> (0:w67:bool)
    n73 = Unbundle By Name(w128) -> ("status"=→"Error Detected":bool)
    n74 = Select(t=w66, s=w67, f=w65) -> (s? t:f=w64:u32)
    n75 = Unbundle By Name(w88) -> ("TC0"=→"TC1":dbl, "TC1"=→"TC2":dbl, "TC2"=→"TC3":dbl, "TC3"=→"TC4":dbl, "TC4"=→"TC5":dbl, "TC5"=→"TC6":dbl)  [unwired: 1 out]
    n76 = Select(t=state-enum."reset", s="Reset", f=w144) -> (s? t:f=w143:T3)
    n77 = call "loop-timer.vi"("loop-time-in"=w124) -> ("Loop Time (mS)"=→"Loop Time (mS)":u32, "loop-time-out"=w123:u32, "Hz"=→"Hz":dbl)  [unwired: 8 in]
    n78 = Select(t=u32 0, s="Reset LD", f=w64) -> (s? t:f=w61:u32)
    "longest delay" <- w61
    n79 = property on="Log Filepath Selection" class="Clust (strict)"("DisabledEnum"=w132) -> ()  [unwired: 2 in, 2 out]
    n80 = Select(t=state-enum."stop", s="Stop ADAM", f=w143) -> (s? t:f=w153:T3)
    n81 = Unbundle By Name(w81) -> ("TC0"=→"TC7":dbl, "TC1"=→"TC8":dbl, "TC2"=→"TC9":dbl, "TC3"=→"TC10":dbl, "TC4"=→"TC11":dbl, "TC5"=→"TC12":dbl)  [unwired: 1 out]
    n82 = Select(t=state-enum."exit", s="exit", f=w153) -> (s? t:f=w156:T3)
    n83 = Or(x=w150, y=w150) -> (x .or. y?=w177:bool)
    n84 = Unbundle By Name(w93) -> ("AI0"=→"P1: Condenser":dbl, "AI1"=→"P2: Adsorber 2":dbl, "AI2"=→"P3: Adsorber 1":dbl, "AI3"=→"P4: Evaporator":dbl)
    n85 = property on="Reset LD" class="Bool"("Visible"="Debug Mode") -> ()  [unwired: 2 in, 2 out]
    n86 = property on="File Open" class="Bool (strict)"("Visible"="Debug Mode") -> ()  [unwired: 2 in, 2 out]
    n87 = property on="Status Indicators" class="Clust (strict)"("Visible"="Debug Mode") -> ()  [unwired: 2 in, 2 out]
    n88 = property on="error" class="Clust (strict)"("Visible"=w177) -> ()  [unwired: 2 in, 2 out]
    n89 = property on="cmd-response" class="Clust (strict)"("Visible"="Debug Mode") -> ()  [unwired: 2 in, 2 out]
    n90 = property on="longest delay" class="DigNum (strict)"("Visible"="Debug Mode") -> ()  [unwired: 2 in, 2 out]
    n91 = property on="Hz" class="DigNum (strict)"("Visible"="Debug Mode") -> ()  [unwired: 2 in, 2 out]
    n92 = property on="Next Log Event mS" class="DigNum (strict)"("Visible"="Debug Mode") -> ()  [unwired: 2 in, 2 out]
    n93 = Wait (ms)(milliseconds to wait=u32 10) -> ()  [unwired: 1 out]
    "Loop Counter" <- w178
    "Program State" <- w139
  }
  n94 = flat-sequence {
    tunnel: w30 -> [w374]
    tunnel: w29 -> [w373]
    tunnel: [w372] -> w28
    tunnel: [w371] -> w27
    tunnel: w11 -> [w370]
    tunnel: [w369] -> w12
    tunnel: w10 -> [w368]
    tunnel: w9 -> [w367]
    tunnel: [w389] -> w33
    tunnel: w28 -> [w388]
    tunnel: w27 -> [w387]
    tunnel: w12 -> [w385]
    tunnel: w33 -> [w395]
    frame #0 {
      (unwired) T12 {"DO0"=FALSE, "DO1"=FALSE, "DO2"=FALSE, "DO3"=FALSE, "DO4"=FALSE, "DO5"=FALSE, "DO6"=FALSE, "DO7"=FALSE} ("5:Digital Outputs")
      n95 = case shown="True" w368 {
        tunnel: w367 -> [_ w376]
        frame False {
        }
        frame True {
          n96 = Close File(refnum=w376) -> (error out=w375:errorcluster)  [unwired: 1 in, 1 out]
          n97 = call <vilib>:"Clear Errors.vi"("error in (no error)"=w375) -> ()  [unwired: 5 in, 2 out]
        }
      }
      n98 = case shown="True" w370 {
        selector: w370 -> [w377 w380]
        tunnel: w374 -> [w379 w384]
        tunnel: w373 -> [w378 w383]
        tunnel: [w378 w382] -> w372
        tunnel: [w379 w381] -> w371
        tunnel: [w377 w380] -> w369
        frame False {
        }
        frame True {
          n99 = call "adam5000-close-all.vi"("VISA Refnum in"=w384, "error in (no error)"=w383) -> ("VISA Refnum out"=w381:refnum<visa-resource-name>, "error out"=w382:errorcluster)  [unwired: 10 in, 2 out]
        }
      }
    }
    frame #1 {
      n100 = case shown="True" w385 {
        tunnel: [w390 w393] -> w389
        tunnel: w388 -> [w390 w392]
        tunnel: w387 -> [_ w391]
        frame False {
        }
        frame True {
          n101 = call "adam5000-stop-visa.vi"("error in (no error)"=w392, "VISA resource in"=w391) -> ("error out"=w393:errorcluster)  [unwired: 9 in]
        }
      }
      n102 = property on="Chassis Settings" class="Clust (strict)"("DisabledEnum"=T17."Enabled" ("Disabled")) -> ()  [unwired: 2 in, 2 out]
    }
    frame #2 {
      n103 = Merge Errors(w395) -> (w394:errorcluster)
      n104 = local write "error"(w394) -> ()
      n105 = Wait (ms)(milliseconds to wait=u32 500) -> ()  [unwired: 1 out]
    }
    frame #3 {
      # "Quit Labview"
      n106 = disable-structure "Conditional Disable Structure" shown="RUN_TIME_ENGINE==True" {
        frame condition #0 (active) {
        }
        frame condition #1 {
          # "Call Quit LabVIEW if running as a built application."
          n107 = Quit LabVIEW() -> ()  [unwired: 1 in]
        }
      }
    }
  }
